vi "IPS120 RH1 - Get Status.vi"(1 "GPIB Address":string="25") -> (0 "Magnet Status":T1={"Sweep Status"=enum."To Zero", "Leads Current (A)"=0.0, "Leads Voltage (V)"=-0.02, "Leads Field (T)"=0.0, "Switch Heater"=FALSE, "Setpoint (A)"=0.0, "Sweep Rate (A/min)"=0.0, "System Status"=enum."Normal", "Limit Status"=enum."Normal", "Persistent Current (A)"=0.0, "Control Status"=FALSE, "Persistent Field (T)"=0.0} {"Leads Field (T)" format="%.3f"; "Persistent Field (T)" format="%.3f"; "Persistent Current (A)" format="%.3f"; "Setpoint (A)" format="%.3f"; "Leads Voltage (V)" format="%.2f"; "Sweep Rate (A/min)" format="%.2f"; "Leads Current (A)" format="%.3f"})   [LabVIEW 2009]
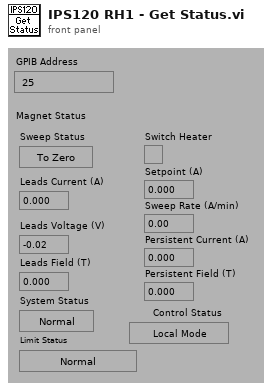
[diagram p1: front panel]
types:
  T1 = cluster{"Sweep Status":enum16{"Hold", "To Setpoint", "To Zero", "Clamped"}, "Leads Current (A)":dbl, "Leads Voltage (V)":dbl, "Leads Field (T)":dbl, "Switch Heater":bool, "Setpoint (A)":dbl, "Sweep Rate (A/min)":dbl, "System Status":enum16{"Normal", "Quenched", "Over Heated", "Warming Up"}, "Limit Status":enum16{"Normal", "Positive Voltage Limit", "Negative Voltage Limit", "Negative Current Limit", "Positive Current Limit"}, "Persistent Current (A)":dbl, "Control Status":bool, "Persistent Field (T)":dbl}
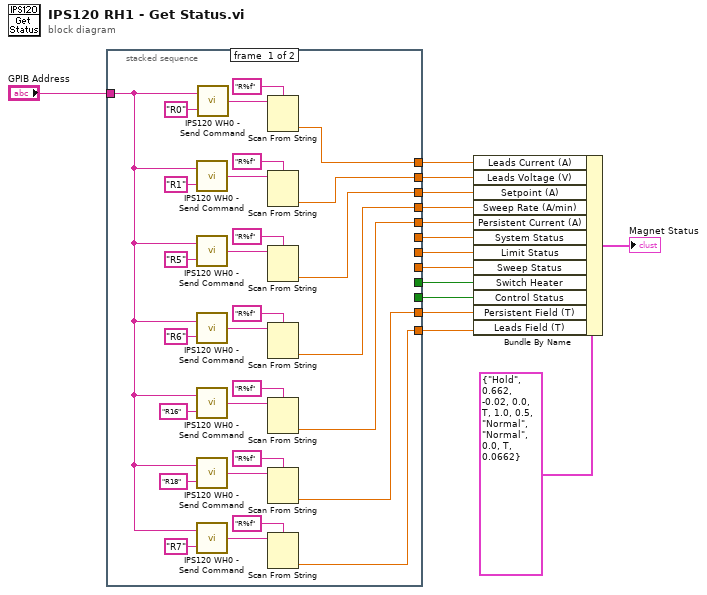
[diagram p0: block diagram]
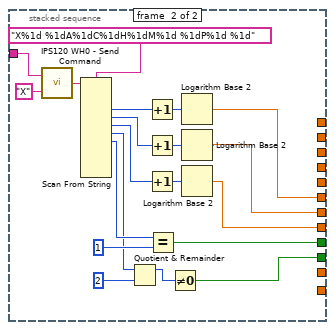
[diagram p2: hidden frame]
diagram:
  n1 = stacked-sequence {
    tunnel: "GPIB Address" -> [w17 w63]
    tunnel: [w44 _] -> w11
    tunnel: [w41 _] -> w12
    tunnel: [w40 _] -> w13
    tunnel: [w39 _] -> w14
    tunnel: [w32 _] -> w15
    tunnel: [_ w58] -> w9
    tunnel: [_ w50] -> w8
    tunnel: [_ w51] -> w7
    tunnel: [_ w52] -> w6
    tunnel: [_ w46] -> w5
    tunnel: [w21 _] -> w4
    tunnel: [w16 _] -> w1
    frame #0 {
      n2 = call "IPS120 WH0 - Send Command.vi"("Command String"="R1", "GPIB Address"=w17) -> ("Response String"=w36:string)
      n3 = call "IPS120 WH0 - Send Command.vi"("Command String"="R5", "GPIB Address"=w17) -> ("Response String"=w37:string)
      n4 = call "IPS120 WH0 - Send Command.vi"("Command String"="R6", "GPIB Address"=w17) -> ("Response String"=w38:string)
      n5 = call "IPS120 WH0 - Send Command.vi"("Command String"="R16", "GPIB Address"=w17) -> ("Response String"=w43:string)
      n6 = call "IPS120 WH0 - Send Command.vi"("Command String"="R18", "GPIB Address"=w17) -> ("Response String"=w22:string)
      n7 = call "IPS120 WH0 - Send Command.vi"("Command String"="R7", "GPIB Address"=w17) -> ("Response String"=w20:string)
      n8 = call "IPS120 WH0 - Send Command.vi"("Command String"="R0", "GPIB Address"=w17) -> ("Response String"=w31:string)
      n9 = Scan From String(format string="R%f", input string=w31) -> (output 1=w32:dbl)  [unwired: 3 in, 3 out]
      n10 = Scan From String(format string="R%f", input string=w36) -> (output 1=w39:dbl)  [unwired: 3 in, 3 out]
      n11 = Scan From String(format string="R%f", input string=w37) -> (output 1=w40:dbl)  [unwired: 3 in, 3 out]
      n12 = Scan From String(format string="R%f", input string=w38) -> (output 1=w41:dbl)  [unwired: 3 in, 3 out]
      n13 = Scan From String(format string="R%f", input string=w43) -> (output 1=w44:dbl)  [unwired: 3 in, 3 out]
      n14 = Scan From String(format string="R%f", input string=w22) -> (output 1=w21:dbl)  [unwired: 3 in, 3 out]
      n15 = Scan From String(format string="R%f", input string=w20) -> (output 1=w16:dbl)  [unwired: 3 in, 3 out]
    }
    frame #1 {
      n16 = call "IPS120 WH0 - Send Command.vi"("Command String"="X", "GPIB Address"=w63) -> ("Response String"=w61:string)
      n17 = Scan From String(format string="X%1d %1dA%1dC%1dH%1dM%1d %1dP%1d %1d", input string=w61) -> (output 1=w60:i32, output 2=w55:i32, output 3=w54:i32, output 4=w48:i32, output 5=w49:i32)  [unwired: 15 in, 3 out]
      n18 = Quotient & Remainder(x=w48, y=2) -> (x-y*floor(x/y)=w45:i32)  [unwired: 1 out]
      n19 = Increment(x=w60) -> (x+1=w59:i32)
      n20 = Increment(x=w55) -> (x+1=w57:i32)
      n21 = Increment(x=w54) -> (x+1=w56:i32)
      n22 = Equal?(x=w49, y=1) -> (x = y?=w52:bool)
      n23 = Not Equal To 0?(x=w45) -> (x != 0?=w46:bool)
      n24 = Logarithm Base 2(1:w59) -> (0:w58:dbl)
      n25 = Logarithm Base 2(1:w57) -> (0:w50:dbl)
      n26 = Logarithm Base 2(1:w56) -> (0:w51:dbl)
    }
  }
  n27 = Bundle By Name(cluster=T1 {"Sweep Status"=enum."Hold", "Leads Current (A)"=0.662, "Leads Voltage (V)"=-0.02, "Leads Field (T)"=0.0, "Switch Heater"=TRUE, "Setpoint (A)"=1.0, "Sweep Rate (A/min)"=0.5, "System Status"=enum."Normal", "Limit Status"=enum."Normal", "Persistent Current (A)"=0.0, "Control Status"=TRUE, "Persistent Field (T)"=0.0662} ("Magnet Status"), "Leads Current (A)"=w15, "Leads Voltage (V)"=w14, "Setpoint (A)"=w13, "Sweep Rate (A/min)"=w12, "Persistent Current (A)"=w11, "System Status"=w9, "Limit Status"=w8, "Sweep Status"=w7, "Switch Heater"=w6, "Control Status"=w5, "Persistent Field (T)"=w4, "Leads Field (T)"=w1) -> (→"Magnet Status":T1)
